vi "Init.vi"(8 "error in (no error)":errorcluster) -> (0 "error out":errorcluster, 3 "Input out":refnum<class "Input.lvclass">)   [LabVIEW 2015, in "Input.lvclass"]
uses:
  Input.lvclass
  Mouse State.ctl
  Input.lvclass/Input.ctl
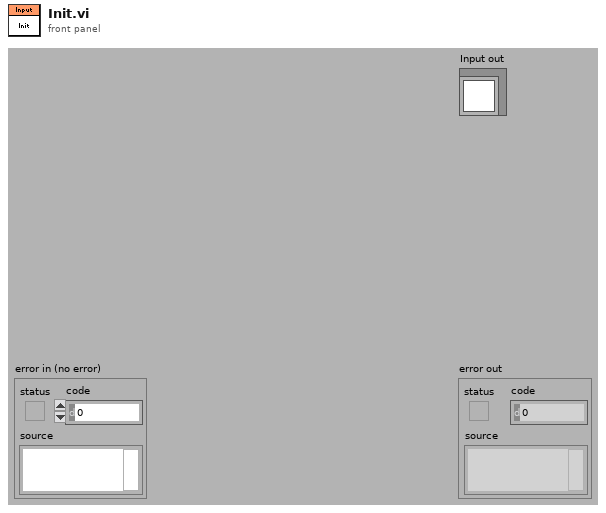
[diagram p1: front panel]
types:
  T1 = typedef "Input.lvclass/Mouse State.ctl" = cluster{"Movement":cluster{"X":i32, "Y":i32, "Scrolling":i32}, "Buttons":cluster{"Button1":bool, "Button2":bool, "Button3":bool, "Button4":bool}}
  T2 = cluster{"Keys Down":enum16{"0", "1", "2", "3", "4", "5", "6", "7", "8", "9", "A", "B", "C", "D", "E", "F", "G", "H", "I", "J", "K", "L", "M", "N", "O", "P", "Q", "R", "S", "T", "U", "V", "W", "X", "Y", "Z", "F1", "F2", "F3", "F4", "F5", "F6", "F7", "F8", "F9", "F10", "F11", "F12", "F13", "F14", "F15", "ADD", "BACK", "BACKSLASH", "CAPITAL", "COMMA", "DECIMAL", "DELETE", "DIVIDE", "DOWN", "END", "EQUALS", "ESCAPE", "GRAVE (`)", "HOME", "INSERT", "LBRACKET", "LCONTROL", "LEFT", "L ALT", "LSHIFT", "LWIN", "MINUS", "MULTIPLY", "NEXT", "NUMLOCK", "NUMPAD_0", "NUMPAD_1", "NUMPAD_2", "NUMPAD_3", "NUMPAD_4", "NUMPAD_5", "NUMPAD_6", "NUMPAD_7", "NUMPAD_8", "NUMPAD_9", "PAUSE", "PERIOD", "PRIOR (PG UP)", "RBRACKET", "RCONTROL", "RETURN", "RIGHT", "R ALT", "RSHIFT", "RWIN", "SCROLL", "SEMICOLON", "SLASH", "SPACE", "SUBTRACT", "TAB", "UP", "ENTER (num pad)", "' (quote)"}[]}
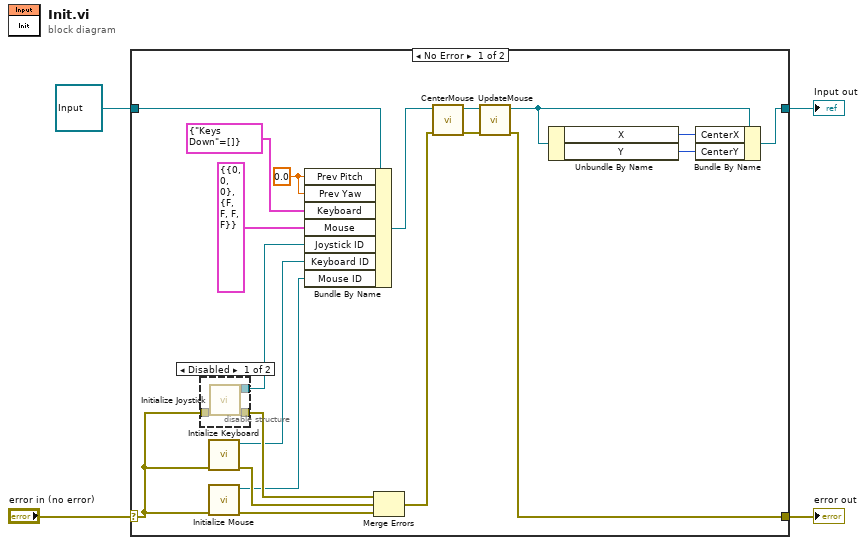
[diagram p0: block diagram]
diagram:
  n1 = case shown="No Error" "error in (no error)" {
    selector: "error in (no error)" -> [w24 w29]
    tunnel: [w5 w29] -> w3
    tunnel: [w10 w28] -> w1
    tunnel: refnum<class "Input.lvclass"> refnum ("Input in") -> [w20 w28]
    frame No Error {
      w13 = sgl 0.0 ("Prev Pitch")
      n2 = disable-structure shown="Disabled" {
        disable-tunnel: w24 -> [w27 _]
        disable-tunnel: [w26 _] -> w23
        disable-tunnel: [w25 _] -> w18
        frame Disabled {
          n3 = call <vilib>:"Initialize Joystick.vi"("error in (no error)"=w27) -> ("error out"=w26:errorcluster, "device ID"=w25:refnum<k1>)  [unwired: 9 in]
        }
        frame Enabled {
        }
      }
      n4 = call <vilib>:"Intialize Keyboard.vi"("error in (no error)"=w24) -> ("error out"=w22:errorcluster, "device ID"=w17:refnum<k1>)  [unwired: 9 in]
      n5 = call <vilib>:"Initialize Mouse.vi"("error in (no error)"=w24) -> ("error out"=w21:errorcluster, "device ID"=w16:refnum<k1>)  [unwired: 9 in]
      n6 = Bundle By Name(cluster=w20, "Prev Pitch"=w13, "Prev Yaw"=w13, "Keyboard"=T2 {"Keys Down"=[]}, "Mouse"=T1 {"Movement"={"X"=0, "Y"=0, "Scrolling"=0}, "Buttons"={"Button1"=FALSE, "Button2"=FALSE, "Button3"=FALSE, "Button4"=FALSE}}, "Joystick ID"=w18, "Keyboard ID"=w17, "Mouse ID"=w16) -> (w15:refnum<class "Input.lvclass">)
      n7 = Merge Errors(w23, w22, w21) -> (w19:errorcluster)
      n8 = call "CenterMouse.vi"("error in (no error)"=w19, "Input in"=w15) -> ("error out"=w9:errorcluster, "Input out"=w11:refnum<class "Input.lvclass">)  [unwired: 8 in]
      n9 = call "UpdateMouse.vi"("error in (no error)"=w9, "Input in"=w11) -> ("error out"=w5:errorcluster, "Input out"=w8:refnum<class "Input.lvclass">)  [unwired: 8 in]
      n10 = Unbundle By Name(w8) -> ("X"=w7:i32, "Y"=w6:i32)
      n11 = Bundle By Name(cluster=w8, "CenterX"=w7, "CenterY"=w6) -> (w10:refnum<class "Input.lvclass">)
    }
    frame Error {
    }
  }
  "error out" <- w3
  "Input out" <- w1
